vi "Get HDI Pad Group Image.vi"(8 "error in":errorcluster, 10 "HDI Pad Group":T1, 11 "CameraTool in":refnum<class "CameraTool Class.lvclass">) -> (0 "error out":errorcluster, 2 "HDI Pad Group Physical Image":T2, 3 "CameraTool out":refnum<class "CameraTool Class.lvclass">)   [LabVIEW 2011, in "CameraTool Class.lvclass"]
uses:
  CameraTool Class.lvclass
  Utils/Type Definitions/Physical Image.ctl
  Vec3d Class/Vec3d Class.lvclass
  <vilib>/vision/Image Controls.llb/IMAQ Image.ctl
  Config Manager Class/Type Definitions/Part Type.ctl
  WorkTable Class/WorkTable Class.lvclass
  Config Manager Class/Read Geometry Definition Integer.vi
  Config Manager Class/Read Geometry Definition Double.vi
  Config Manager Class/Read Geometry Definition 3D.vi
  Config Manager Class/Config Manager Class.lvclass
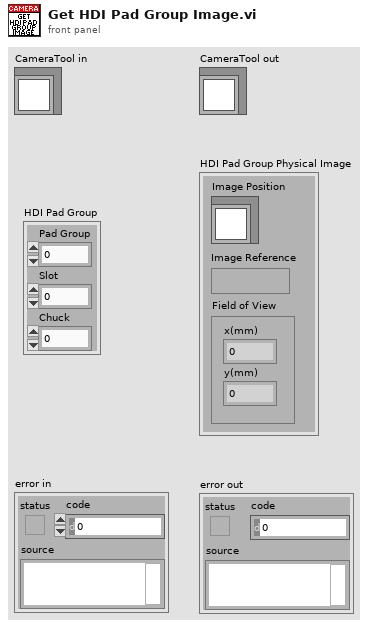
[diagram p1: front panel]
types:
  T1 = cluster{"Pad Group":i32, "Slot":i32, "Chuck":i32}
  T2 = typedef "Physical Image.ctl" = cluster{"Image Position":refnum<class "Vec3d Class.lvclass">, "Image Reference":T3, "Field of View":cluster{"x(mm)":dbl, "y(mm)":dbl}}
  T3 = typedef "IMAQ Image.ctl" = refnum<image>
  T4 = typedef "Part Type.ctl" = enum16{"BBM", "HDI", "BARE HDI", "GLUERESERVOIR", "STAMP_1", "STAMP_2", "STAMP_3", "STAMP_4", "STAMP_5", "WEIGHT_1", "WEIGHT_2", "WEIGHT_3", "WEIGHT_4", "WEIGHT_5", "WEIGHT_6", "WEIGHT_7", "WEIGHT_8", "PICKER_TOOL", "GRABER_TOOL"}
  T5 = typedef "Worktable_Module Slot.ctl" = cluster{"Slot State":enum16{"Empty", "Bare HDI", "Unglued", "Stamped", "PartOnTop", "Weighted", "Unpotted", "Potted"}, "BBM Type":enum16{"None", "BBM", "GlassSlide"}, "HDI Type":enum16{"None", "HDI", "Polyimide"}, "Vacuum Channel":u8, "Location/Orientation BBM":T6, "Location/Orientation HDI":T6, "S/N":string}
  T6 = typedef "Position_Orientation.ctl" = cluster{"Center":refnum<class "Vec3d Class.lvclass">, "Orientation":refnum<class "Orient3d Class.lvclass">}
  T7 = typedef "3d Line.ctl" = cluster{"Start":refnum<class "Vec3d Class.lvclass">, "End":refnum<class "Vec3d Class.lvclass">, "Enable":bool}
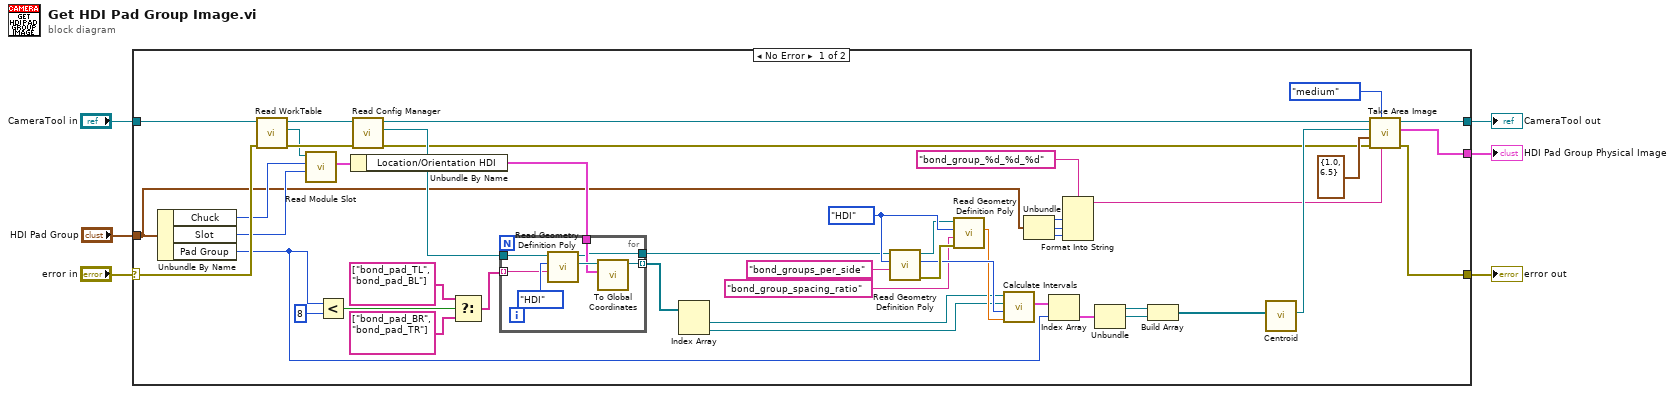
[diagram p0: block diagram]
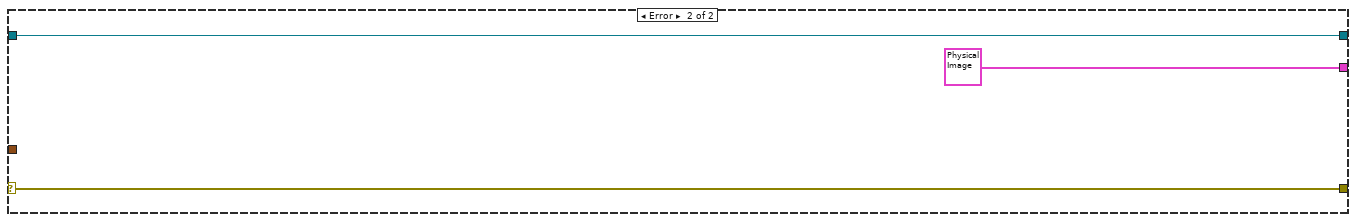
[diagram p2: hidden frame]
diagram:
  n1 = case shown="No Error" "error in" {
    selector: "error in" -> [w49 w62]
    tunnel: [w14 T2 {"Image Position"=refnum, "Image Reference"=refnum, "Field of View"={"x(mm)"=0.0, "y(mm)"=0.0}} ("Composite Physical Image")] -> w6
    tunnel: [w13 w61] -> w5
    tunnel: [w12 w62] -> w4
    tunnel: "CameraTool in" -> [w52 w61]
    tunnel: "HDI Pad Group" -> [w18 _]
    frame No Error {
      w30 = Part_Type."HDI" ("Part Type")
      n2 = Unbundle By Name(w18) -> ("Chuck"=w45:i32, "Slot"=w46:i32, "Pad Group"=w23:i32)
      n3 = call-dynamic "Read WorkTable.vi"("error in"=w49, "Gantry Class in"=w52) -> ("error out"=w50:errorcluster, "WorkTable Class.lvclass"=w48:refnum<class "WorkTable Class.lvclass">, "Gantry Class out"=w51:refnum<class "CameraTool Class.lvclass">)  [unwired: 7 in]
      n4 = call-dynamic "Read Module Slot.vi"("slot"=w46, "chuck"=w45, "WorkTable in"=w48) -> ("Module Slot"=w47:T5)  [unwired: 6 in, 2 out]
      n5 = Less?(x=w23, y=8) -> (x < y?=w41:bool)
      n6 = Unbundle By Name(w47) -> ("Location/Orientation HDI"=w38:T6)
      n7 = call-dynamic "Read Config Manager.vi"("error in"=w50, "Gantry in"=w51) -> ("error out"=w19:errorcluster, "Config Manager"=w40:refnum<class "Config Manager Class.lvclass">, "Gantry out"=w37:refnum<class "CameraTool Class.lvclass">)  [unwired: 7 in]
      n8 = Select(t=string[] ["bond_pad_TL", "bond_pad_BL"], s=w41, f=string[] ["bond_pad_BR", "bond_pad_TR"]) -> (s? t:f=w39:string[])
      n9 = for {
        tunnel: w40 -> [w54]
        tunnel: w39 -> [w58] mode=indexing
        tunnel: w38 -> [w56]
        tunnel: [w55] -> w27 mode=indexing
        tunnel: [w53] -> w28
        n10 = call-poly "Read Geometry Definition Poly.vi"("Feature"=w58, "Part Type"=Part_Type."HDI", "Config Manager in"=w54) -> ("Feature Coordinates"=w57:refnum<class "Vec3d Class.lvclass">, "Config Manager out"=w53:refnum<class "Config Manager Class.lvclass">)  [unwired: 6 in, 1 out]
        n11 = call "To Global Coordinates.vi"("Center/Orientation"=w56, "Local Coordinates"=w57) -> ("Global Coordinates"=w55:refnum<class "Vec3d Class.lvclass">)  [unwired: 8 in, 1 out]
      }
      n12 = Index Array(array=w27) -> (element #1=w26:refnum<class "Vec3d Class.lvclass">, element #2=w25:refnum<class "Vec3d Class.lvclass">)  [unwired: 2 in]
      n13 = call-poly "Read Geometry Definition Poly.vi"("Feature"="bond_groups_per_side", "Part Type"=w30, "Config Manager in"=w28) -> ("error out"=w35:errorcluster, "Geometry Definition"=w34:i32, "Config Manager out"=w29:refnum<class "Config Manager Class.lvclass">)  [unwired: 6 in]
      n14 = call-poly "Read Geometry Definition Poly.vi"("error in"=w35, "Feature"="bond_group_spacing_ratio", "Part Type"=w30, "Config Manager in"=w29) -> ("Geometry Definition"=w33:dbl)  [unwired: 5 in, 2 out]
      n15 = call "Calculate Intervals.vi"("gap/group ratio"=w33, "Num Intervals"=w34, "End"=w25, "Start"=w26) -> ("Intervals"=w24:T7[])  [unwired: 7 in]
      n16 = Unbundle(w18) -> ("Pad Group"=w17:i32, "Slot"=w16:i32, "Chuck"=w15:i32)
      n17 = Index Array(array=w24, index=w23) -> (element=w11:T7)
      n18 = Format Into String(format string="bond_group_%d_%d_%d", w17, w16, w15) -> (resulting string=w20:string)  [unwired: 2 in, 1 out]
      n19 = Unbundle(w11) -> ("Start"=w10:refnum<class "Vec3d Class.lvclass">, "End"=w9:refnum<class "Vec3d Class.lvclass">)  [unwired: 1 out]
      n20 = Build Array(w10, w9) -> (w8:refnum<class "Vec3d Class.lvclass">[])
      n21 = call "Centroid.vi"("Points"=w8) -> ("Centroid"=w22:refnum<class "Vec3d Class.lvclass">)  [unwired: 10 in]
      n22 = call "Take Area Image.vi"("Image Name"=w20, "Quality"=enum16{"perfect", "high", "medium", "low"}."medium", "error in"=w19, "Field of View"=cluster{"Size-X(mm)":dbl, "Size-Y(mm)":dbl} {"Size-X(mm)"=1.0, "Size-Y(mm)"=6.5}, "Image Center"=w22, "CameraTool in"=w37) -> ("error out"=w12:errorcluster, "Physical Image"=w14:T2, "CameraTool out"=w13:refnum<class "CameraTool Class.lvclass">)  [unwired: 3 in]
    }
    frame Error {
    }
  }
  "HDI Pad Group Physical Image" <- w6
  "error out" <- w4
  "CameraTool out" <- w5
